vi "ESR Processing.vi"(9 "ESR Post-Processing Parameters":T1={"Cut-off Threshhold"=1.3, "Processing Type"=enum."Off"}, 10 "Array":u32[][](array[numeric]), 11 "Flourescence Data in":i32[][](array[numeric])) -> (3 "Flourescence Data out":i32[][](array[numeric]))   [LabVIEW 2012]
uses:
  ESR Processing Params.ctl
  ESR Processing State.ctl
  <vilib>/Analysis/baseanly.llb/Mean (DBL).vi
  <vilib>/Analysis/NI_AALBase.lvlib
panel:
  # "* <data>"
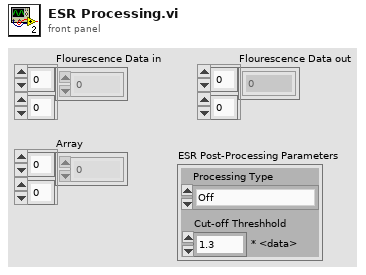
[diagram p1: front panel]
types:
  T1 = typedef "ESR Processing Params.ctl" = cluster{"Cut-off Threshhold":dbl, "Processing Type":T2}
  T2 = typedef "ESR Processing State.ctl" = enum16{"Off", "Remove Outlier Scan", "Remove Outlier Data"}
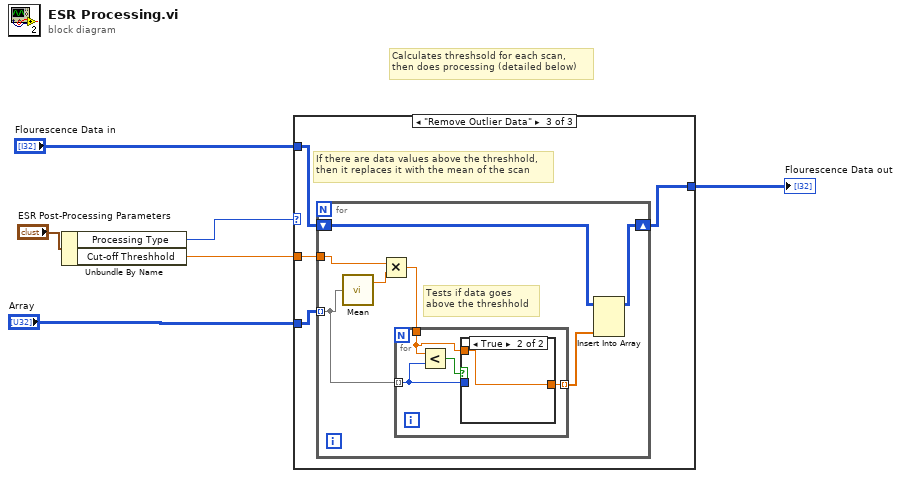
[diagram p0: block diagram]
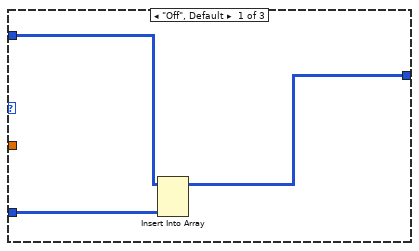
[diagram p2: hidden frame]
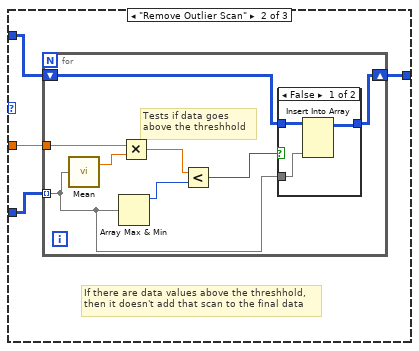
[diagram p3: hidden frame]
diagram:
  # "Calculates threshsold for each scan,\nthen does processing (detailed below)"
  n1 = Unbundle By Name("ESR Post-Processing Parameters") -> ("Processing Type"=w2:T2, "Cut-off Threshhold"=w1:dbl)
  n2 = case shown="\"Remove Outlier Data\"" w2 {
    tunnel: [w9 w10 w26] -> w6
    tunnel: "Array" -> [w8 w13 w27]
    tunnel: "Flourescence Data in" -> [w7 w11 w29]
    tunnel: w1 -> [_ w12 w28]
    frame "Off", Default {
      n3 = Insert Into Array(array=w7, new element=w8) -> (w9:i32[][])  [unwired: 2 in]
    }
    frame "Remove Outlier Scan" {
      # "If there are data values above the threshhold,\nthen it doesn't add that scan to the final data"
      n4 = for {
        tunnel: w13 -> [w15] mode=indexing
        tunnel: w12 -> [w20]
        shift-right: [w14] -> w10
        shift-left: w11 -> [w16]
        # "Tests if data goes\nabove the threshhold"
        n5 = call-poly <vilib>:"Mean.vi"("X"=w15) -> ("mean"=w21:dbl)  [unwired: 1 out]
        n6 = Array Max & Min(array=w15) -> (max value=w18:u32)  [unwired: 3 out]
        n7 = Multiply(x=w20, y=w21) -> (x*y=w19:dbl)
        n8 = Less?(x=w19, y=w18) -> (x < y?=w17:bool)
        n9 = case shown="False" w17 {
          tunnel: w16 -> [w23 w25]
          tunnel: [w24 w25] -> w14
          tunnel: w15 -> [w22 _]
          frame False {
            n10 = Insert Into Array(array=w23, new element=w22) -> (w24:i32[][])  [unwired: 2 in]
          }
          frame True {
          }
        }
      }
    }
    frame "Remove Outlier Data" {
      # "If there are data values above the threshhold,\nthen it replaces it with the mean of the scan"
      n11 = for {
        tunnel: w27 -> [w34] mode=indexing
        tunnel: w28 -> [w35]
        shift-right: [w30] -> w26
        shift-left: w29 -> [w31]
        # "Tests if data goes\nabove the threshhold"
        n12 = call-poly <vilib>:"Mean.vi"("X"=w34) -> ("mean"=w36:dbl)  [unwired: 1 out]
        n13 = Multiply(x=w35, y=w36) -> (x*y=w33:dbl)
        n14 = for {
          tunnel: w34 -> [w39] mode=indexing
          tunnel: w33 -> [w37]
          tunnel: [w38] -> w32 mode=indexing
          n15 = Less?(x=w37, y=w39) -> (x < y?=w40:bool)
          n16 = case shown="True" w40 {
            tunnel: [w41 w42] -> w38
            tunnel: w39 -> [w41 _]
            tunnel: w37 -> [_ w42]
            frame False {
            }
            frame True {
            }
          }
        }
        n17 = Insert Into Array(array=w31, new element=w32) -> (w30:i32[][])  [unwired: 2 in]
      }
    }
  }
  "Flourescence Data out" <- w6
